vi "DIO run.vi"(0 "FPGA VI Reference In":refnum<k20>, 5 "error in":errorcluster) -> (7 "real-time port A monitor":bool[](array[boolean]), 9 "real-time port B monitor":bool[](array[boolean]), 11 "real-time port C monitor":bool[](array[boolean]), 13 "real-time port D monitor":bool[](array[boolean]), 14 "FPGA VI Reference Out":refnum<k20>, 16 "Time elapsed":dbl, 19 "error out":errorcluster)   [LabVIEW 2017]
uses:
  <vilib>/Utility/error.llb/Error Cluster From Error Code.vi
  <vilib>/rvi/errors/niLvFpgaAdjustHostInterfaceError.vi
  <vilib>/rvi/interface/nirviReadWriteControl/nirviReadWriteControl.xnode
  <vilib>/rvi/interface/Simulation/niFpgaSimulationCallBeginRW.vi
  NiFpgaLv.dll
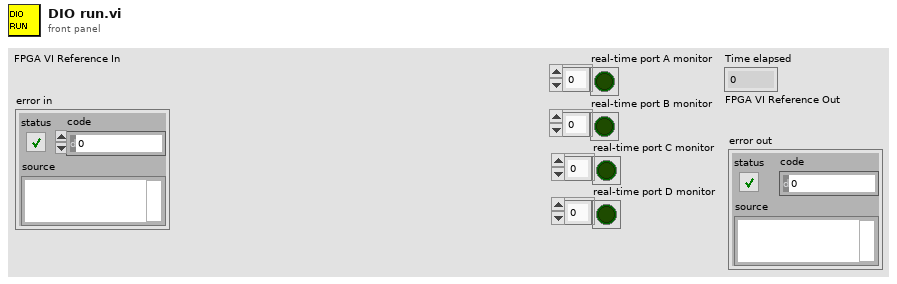
[diagram p1: front panel]
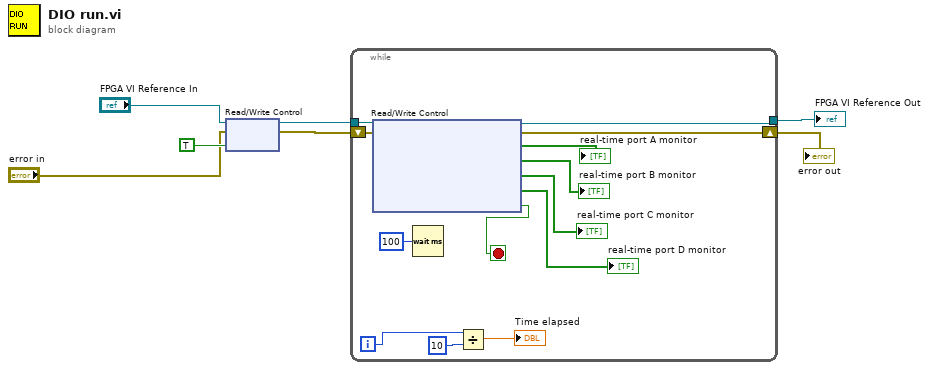
[diagram p0: block diagram]
diagram:
  n1 = xnode "Read/Write Control"("FPGA VI Reference In"="FPGA VI Reference In", "error in"="error in", "Run"=TRUE) -> ("FPGA VI Reference Out"=w4:refnum<k20>, "error out"=w3:errorcluster)
  n2 = while {
    tunnel: w4 -> [w20]
    shift-right: [w14] -> w1
    shift-left: w3 -> [w19]
    tunnel: [w13] -> w2
    i -> [w10]
    stop <- w8 stop-if-true
    n3 = xnode "Read/Write Control"("FPGA VI Reference In"=w20, "error in"=w19) -> ("FPGA VI Reference Out"=w13:refnum<k20>, "error out"=w14:errorcluster, "real-time port A monitor"=→"real-time port A monitor":bool[], "real-time port B monitor"=→"real-time port B monitor":bool[], "real-time port C monitor"=→"real-time port C monitor":bool[], "real-time port D monitor"=→"real-time port D monitor":bool[], "idle LED"=w8:bool)
    n4 = Wait (ms)(milliseconds to wait=u32 100) -> ()  [unwired: 1 out]
    n5 = Divide(x=w10, y=10) -> (x/y=→"Time elapsed":dbl)
  }
  "FPGA VI Reference Out" <- w2
  "error out" <- w1
